vi "电源管理UI.vi"() -> ()   [LabVIEW 2016, in "PLC.lvlib"]
uses:
  PLC.lvlib
  <vilib>/Utility/miscctls.llb/LVPointTypeDef.ctl
panel:
  out "CODCr空闲时间":dbl caption="空闲时间:"
  out "总磷总氮空闲时间":dbl caption="空闲时间:"
  out "营养盐空闲时间":dbl caption="空闲时间:"
  out "CODMn空闲时间":dbl caption="空闲时间:"
  out "多参数空闲时间":dbl caption="空闲时间:"
  in  "CODCr电源":bool
  in  "总磷总氮电源":bool
  in  "营养盐电源":bool
  in  "CODMn电源":bool
  in  "多参数电源":bool
  # "说明：\n系统模式处于维护模式时，仪器电源自动打开；\n系统模式处于常规模式/质控模式/应急模式下，周期启动时，仪器电源自动打开；"
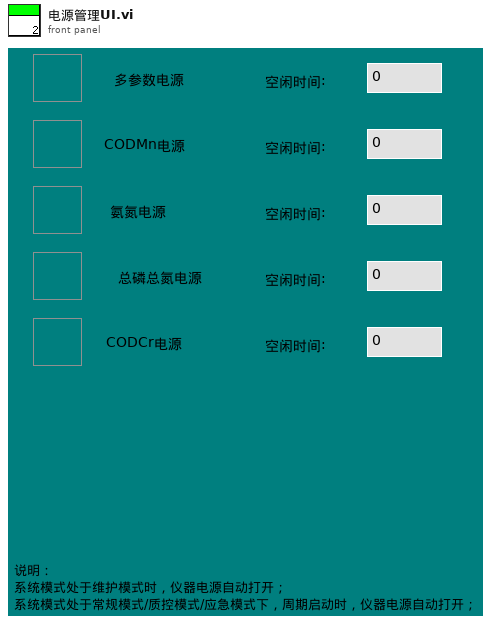
[diagram p1: front panel]
types:
  T1 = typedef "LVPointTypeDef.ctl" = cluster{"Horizontal":i16, "Vertical":i16}
  T2 = enum16{"空闲", "水样测试", "标样核查", "零点核查", "跨度核查", "空白测试", "平行样测试", "加标回收", "空白校准", "标样校准", "初始化（清洗）"}
  T3 = cluster{"R0":i16, "R1":i16, "R2":i16, "R3":i16, "R4":i16, "R5":i16, "R6":i16, "R7":i16, "R8":i16, "R9":i16, "R10":i16, "R11":i16, "R12":i16, "R13":i16, "R14":i16, "R15":i16, "R16":i16, "R17":i16, "R18":i16, "R19":i16, "R20":i16, "R21":i16, "R22":i16, "R23":i16, "R24":i16, "R25":i16, "R26":i16, "R27":i16, "R28":i16, "R29":i16, "R30":i16, "R31":i16, "R32":i16, "R33":i16, "R34":i16, "R35":i16, "R36":i16, "R37":i16, "R38":i16, "R39":i16, "R40":i16, "R41":i16, "R42":i16, "R43":i16, "R44":i16, "R45":i16, "R46":i16, "R47":i16, "R48":i16, "R49":i16, "R50":i16, "R51":i16, "R52":i16, "R53":i16, "R54":i16, "R55":i16, "R56":i16}
  T4 = cluster{"系统时间":timestamp, "工作状态":enum16{"空闲", "水样测试", "标样核查", "零点核查", "跨度核查", "空白测试", "平行样测试", "加标回收", "空白校准", "标样校准", "初始化（清洗）"}, "测量模式":enum16{"待机", "连续模式", "周期模式", "定点模式", "受控模式", "手动模式"}, "告警代码":enum16{"无告警", "缺试剂告警", "缺水样告警", "缺蒸馏水告警", "缺标液告警", "仪表漏液告警", "标定异常告警", "超量程告警", "加热异常", "低试剂预警", "超上限告警", "超下限告警", "仪表内部其他异常", "滴定异常告警", "电极异常告警", "量程切换告警", "参数设置告警", "PH电极电位异常", "电导率电极异常", "浊度光度异常", "溶解氧电极异常", "溶解氧光强异常", "温度异常告警", "PH异常告警", "溶解氧异常告警", "电导率异常告警", "浊度异常告警", "叶绿素异常告警", "藻密度异常告警", "蓝绿藻异常告警", "ORP异常告警", "氨氮异常告警", "清洁刷异常告警", "SD卡异常告警", "蓝牙异常告警", "Wifi异常告警", "流程异常告警"}, "故障代码":enum16{"无故障", "电机故障", "温度故障", "通讯故障", "滴定故障"}, "日志代码":u16, "软件版本":u16, "F0":sgl, "F1":sgl, "F2":sgl, "F3":sgl, "T":sgl, "H":sgl, "id":u16, "flowid":u16, "量程":u16, "总磷控温温度1":sgl, "营养盐控温温度2":sgl, "ADC":sgl}
  T5 = cluster{"系统时间":timestamp, "工作状态":u16, "测量模式":u16, "告警代码":enum16{"无告警", "缺试剂告警", "缺水样告警", "缺蒸馏水告警", "缺标液告警", "仪表漏液告警", "标定异常告警", "超量程告警", "加热异常", "低试剂预警", "超上限告警", "超下限告警", "仪表内部其他异常", "滴定异常告警", "电极异常告警", "量程切换告警", "参数设置告警", "PH电极电位异常", "电导率电极异常", "浊度光度异常", "溶解氧电极异常", "溶解氧光强异常", "温度异常告警", "PH异常告警", "溶解氧异常告警", "电导率异常告警", "浊度异常告警", "叶绿素异常告警", "藻密度异常告警", "蓝绿藻异常告警", "ORP异常告警", "氨氮异常告警", "清洁刷异常告警", "SD卡异常告警", "蓝牙异常告警", "Wifi异常告警", "流程异常告警"}, "故障代码":enum16{"无故障", "电机故障", "温度故障", "通讯故障", "滴定故障"}, "日志代码":u16, "软件版本":string}
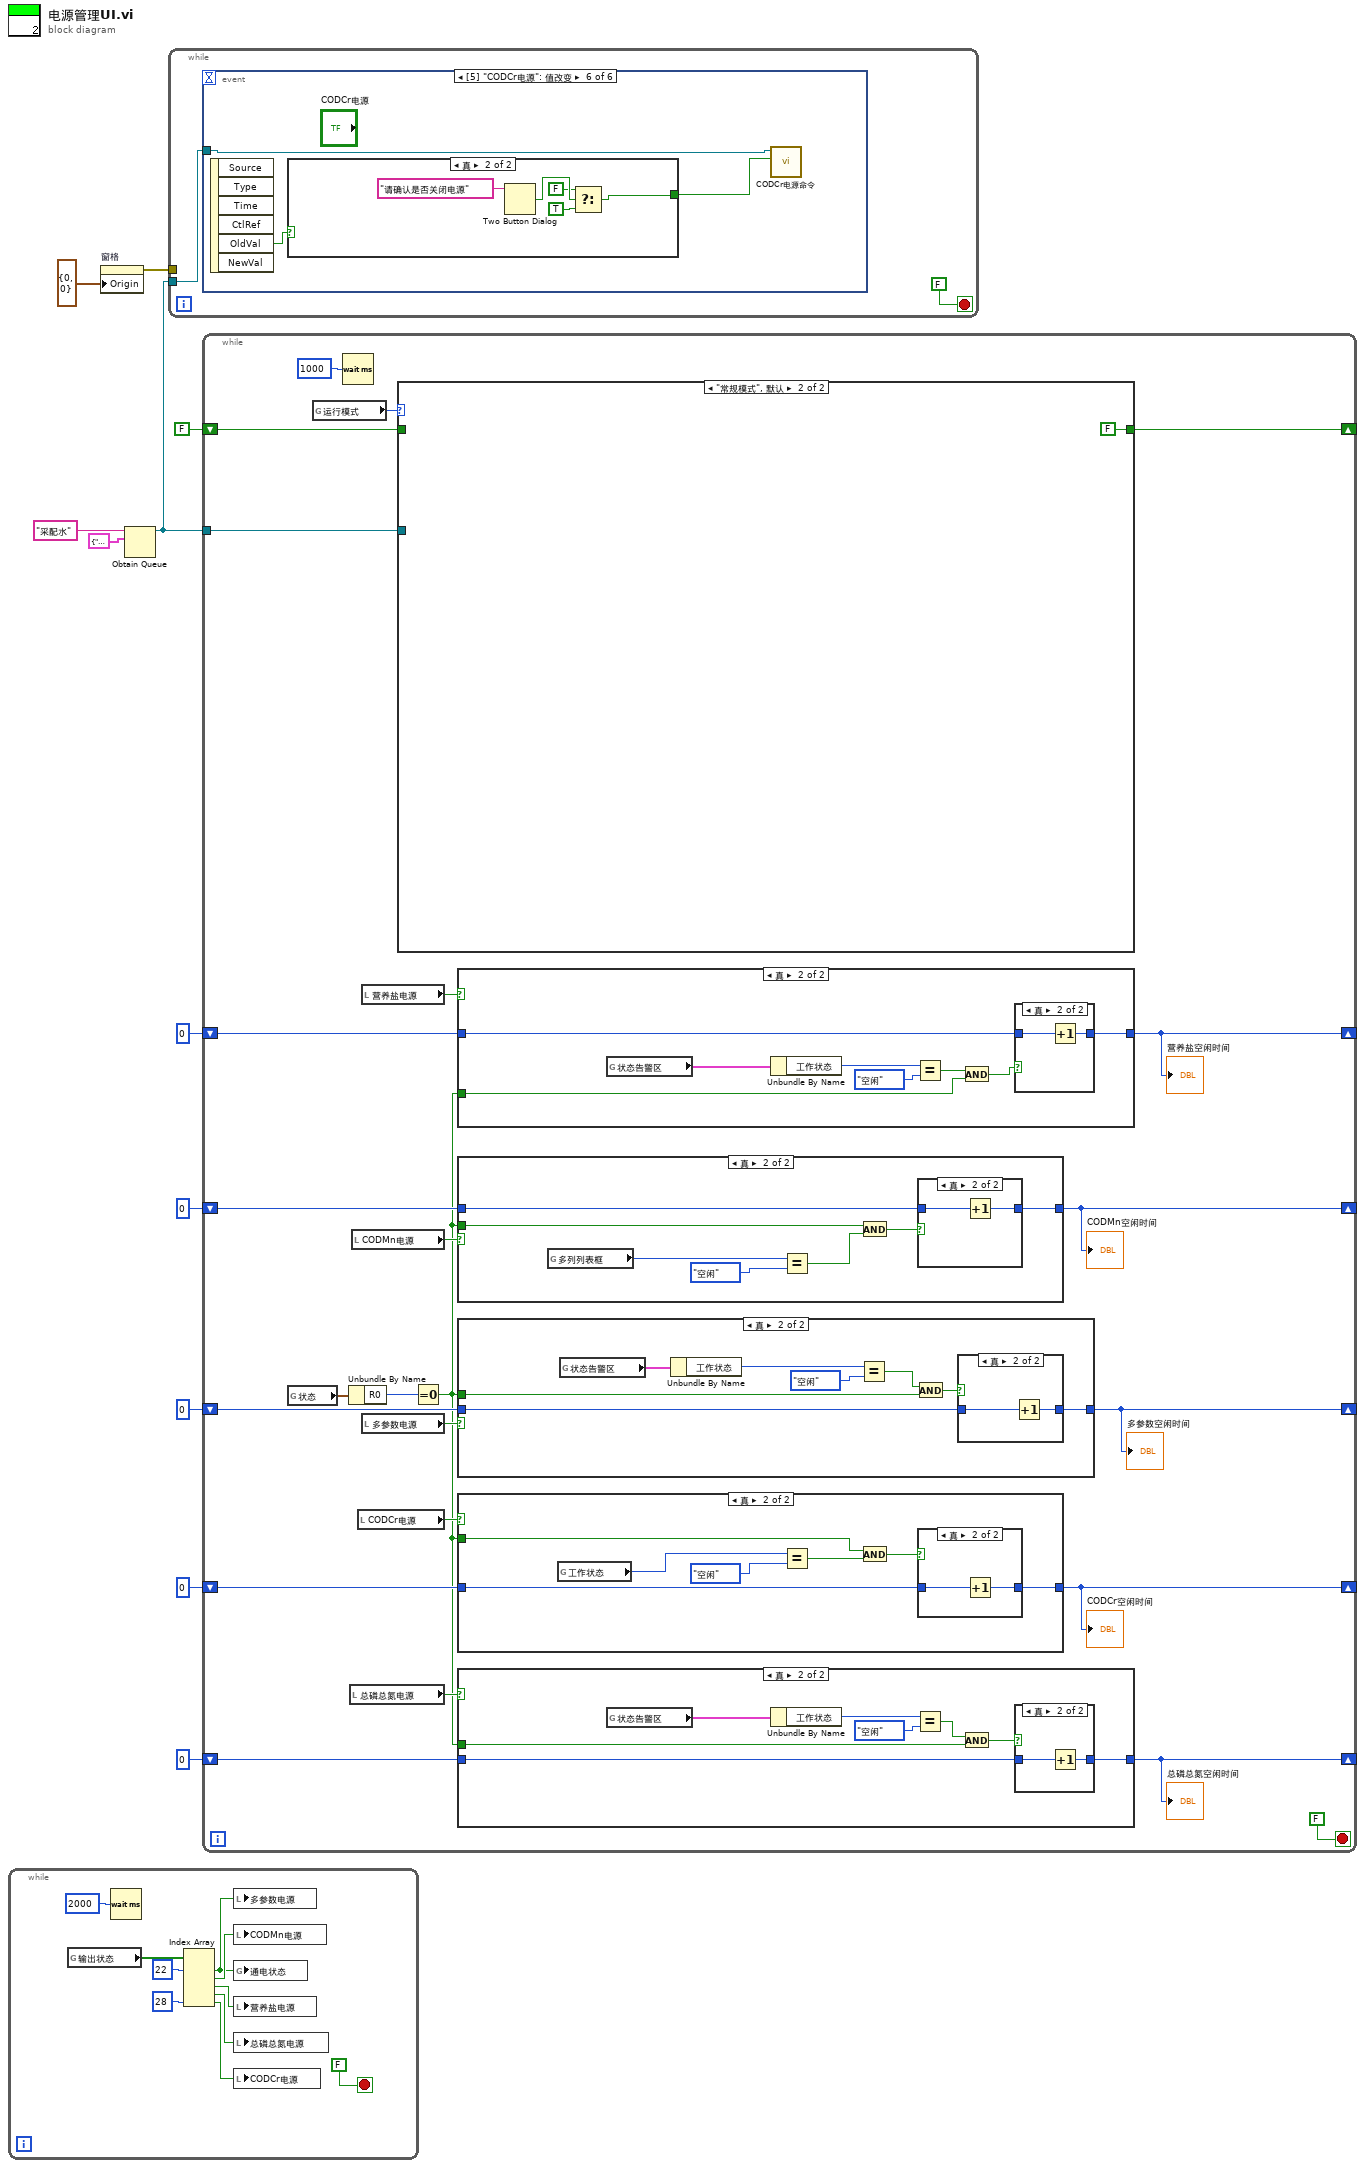
[diagram p0: block diagram]
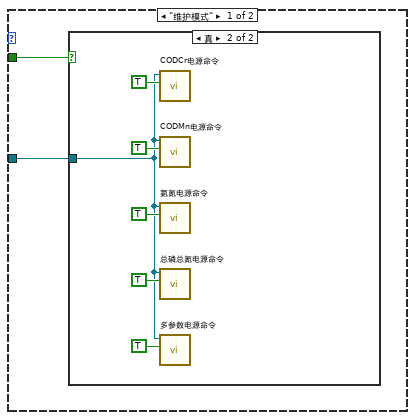
[diagram p2: hidden frame]
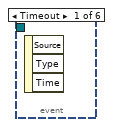
[diagram p14: hidden frame]
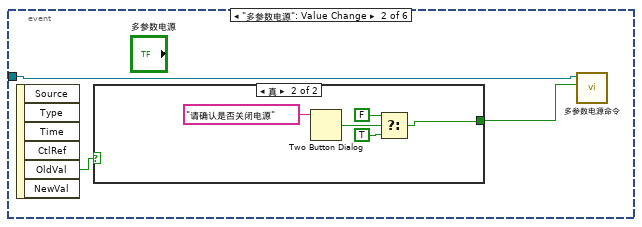
[diagram p15: hidden frame]
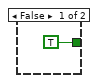
[diagram p16: hidden frame]
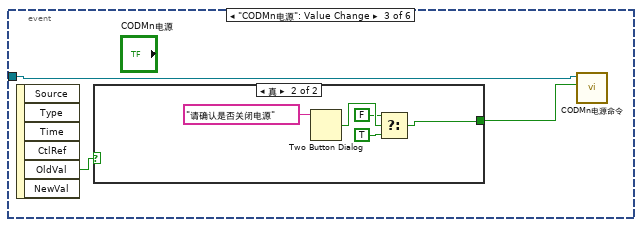
[diagram p17: hidden frame]
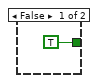
[diagram p18: hidden frame]
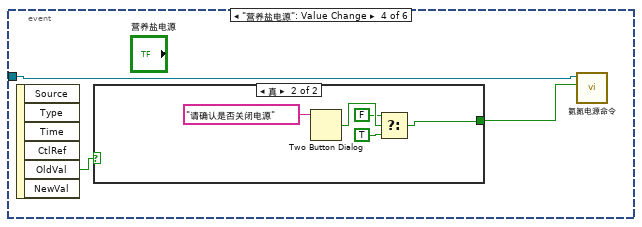
[diagram p19: hidden frame]
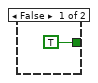
[diagram p20: hidden frame]
diagram:
  n1 = while {
    stop <- FALSE stop-if-true
    n2 = global read "采配水全局变量.vi" "输出状态"() -> (w19:bool[])
    n3 = Wait (ms)(milliseconds to wait=u32 2000 ("等待时间（毫秒）")) -> ()  [unwired: 1 out]
    n4 = Index Array(array=w19, index #1=22 ("索引"), index #5=28 ("索引")) -> (element #1=w14:bool, element #2=w17:bool, element #3=w16:bool, element #4=w15:bool, element #5=w13:bool)  [unwired: 3 in]
    n5 = local write "多参数电源"(w14) -> ()
    n6 = local write "CODMn电源"(w17) -> ()
    n7 = global write "多参数全局变量.vi" "通电状态"(w14) -> ()
    n8 = local write "营养盐电源"(w16) -> ()
    n9 = local write "总磷总氮电源"(w15) -> ()
    n10 = local write "CODCr电源"(w13) -> ()
  }
  n11 = property on="窗格" class="Pane"("Origin"=T1 {"Horizontal"=0, "Vertical"=0} ("原点")) -> (error out=w8:errorcluster)  [unwired: 2 in, 1 out]
  n12 = Obtain Queue(name (unnamed)="采配水" ("名称（未命名）"), element data type=cluster{"命令":string, "数据":variant} {"命令"="", "数据"=variant}) -> (queue out=w7:refnum<queue>)  [unwired: 3 in, 2 out]
  n13 = while {
    tunnel: w7 -> [w22]
    tunnel: w8 -> [_]
    stop <- FALSE stop-if-true
    n14 = event shown="[5] \"CODCr电源\": 值改变" {
      selector: _ -> [_ _ _ _ _ _]
      dyn-events: _ -> [_ _ _ _ _ _]
      timeout: _ -> [_ _ _ _ _ _]
      tunnel: w22 -> [_ w26 w35 w44 w53 w62]
      event Timeout {
        n15 = event-data() -> ()  [unwired: 1 in, 3 out]
      }
      event "多参数电源": Value Change {
        n16 = event-data() -> ("OldVal"=w25:bool)  [unwired: 1 in, 5 out]
        n17 = case shown="真" w25 {
          tunnel: [TRUE ("T button?") w28] -> w24
          frame False {
          }
          frame True {
            n18 = Two Button Dialog(message="请确认是否关闭电源" ("消息")) -> (T button?=w31:bool)  [unwired: 2 in]
            n19 = Select(t=FALSE, s=w31, f=TRUE ("T button?")) -> (s? t:f=w28:bool)
          }
        }
        n20 = call "多参数电源命令.vi"("通电/断电"=w24, "队列"=w26) -> ()  [unwired: 9 in, 1 out]
      }
      event "CODMn电源": Value Change {
        n21 = event-data() -> ("OldVal"=w34:bool)  [unwired: 1 in, 5 out]
        n22 = case shown="真" w34 {
          tunnel: [TRUE ("T button?") w37] -> w33
          frame False {
          }
          frame True {
            n23 = Two Button Dialog(message="请确认是否关闭电源" ("消息")) -> (T button?=w40:bool)  [unwired: 2 in]
            n24 = Select(t=FALSE, s=w40, f=TRUE ("T button?")) -> (s? t:f=w37:bool)
          }
        }
        n25 = call "CODMn电源命令.vi"("通电/断电"=w33, "队列"=w35) -> ()  [unwired: 9 in, 1 out]
      }
      event "营养盐电源": Value Change {
        n26 = event-data() -> ("OldVal"=w43:bool)  [unwired: 1 in, 5 out]
        n27 = case shown="真" w43 {
          tunnel: [TRUE ("T button?") w46] -> w42
          frame False {
          }
          frame True {
            n28 = Two Button Dialog(message="请确认是否关闭电源" ("消息")) -> (T button?=w49:bool)  [unwired: 2 in]
            n29 = Select(t=FALSE, s=w49, f=TRUE ("T button?")) -> (s? t:f=w46:bool)
          }
        }
        n30 = call "氨氮电源命令.vi"("通电/断电"=w42, "队列"=w44) -> ()  [unwired: 9 in, 1 out]
      }
      event "总磷总氮电源": Value Change {
        n31 = event-data() -> ("OldVal"=w52:bool)  [unwired: 1 in, 5 out]
        n32 = case shown="真" w52 {
          tunnel: [TRUE ("T button?") w55] -> w51
          frame False {
          }
          frame True {
            n33 = Two Button Dialog(message="请确认是否关闭电源" ("消息")) -> (T button?=w58:bool)  [unwired: 2 in]
            n34 = Select(t=FALSE, s=w58, f=TRUE ("T button?")) -> (s? t:f=w55:bool)
          }
        }
        n35 = call "总磷总氮电源命令.vi"("通电/断电"=w51, "队列"=w53) -> ()  [unwired: 9 in, 1 out]
      }
      event "CODCr电源": Value Change {
        n36 = event-data() -> ("OldVal"=w61:bool)  [unwired: 1 in, 5 out]
        n37 = case shown="真" w61 {
          tunnel: [TRUE ("T button?") w64] -> w60
          frame False {
          }
          frame True {
            n38 = Two Button Dialog(message="请确认是否关闭电源" ("消息")) -> (T button?=w67:bool)  [unwired: 2 in]
            n39 = Select(t=FALSE, s=w67, f=TRUE ("T button?")) -> (s? t:f=w64:bool)
          }
        }
        n40 = call "CODCr电源命令.vi"("通电/断电"=w60, "队列"=w62) -> ()  [unwired: 9 in, 1 out]
      }
    }
  }
  n41 = while {
    tunnel: w7 -> [w75]
    shift-right: [w76] -> _
    shift-left: u32 0 ("等待时间（毫秒）") -> [w89]
    shift-right: [w80] -> _
    shift-left: u32 0 ("等待时间（毫秒）") -> [w87]
    shift-right: [w78] -> _
    shift-left: u32 0 ("等待时间（毫秒）") -> [w83]
    shift-right: [w79] -> _
    shift-left: u32 0 ("等待时间（毫秒）") -> [w84]
    shift-right: [w77] -> _
    shift-left: u32 0 ("等待时间（毫秒）") -> [w82]
    shift-right: [w72] -> _
    shift-left: FALSE -> [w73]
    stop <- FALSE stop-if-true
    n42 = global read "采配水全局变量.vi" "状态"() -> (w71:T3)
    n43 = global read "系统变量.vi" "运行模式"() -> (w74:enum16{"维护模式", "常规模式", "应急模式", "质控模式"})
    n44 = Wait (ms)(milliseconds to wait=u32 1000 ("等待时间（毫秒）")) -> ()  [unwired: 1 out]
    n45 = Unbundle By Name(w71) -> ("R0"=w70:i16)
    n46 = local read "总磷总氮电源"() -> (w86:bool)
    n47 = local read "CODMn电源"() -> (w88:bool)
    n48 = local read "CODCr电源"() -> (w81:bool)
    n49 = local read "营养盐电源"() -> (w90:bool)
    n50 = local read "多参数电源"() -> (w85:bool)
    n51 = case shown="\"常规模式\", 默认" w74 {
      tunnel: w75 -> [w94 _]
      tunnel: w73 -> [w93 _]
      tunnel: [_ FALSE] -> w72
      frame "维护模式" {
        n52 = case shown="真" w93 {
          tunnel: w94 -> [_ w95]
          frame False {
          }
          frame True {
            n53 = call "CODCr电源命令.vi"("通电/断电"=TRUE, "队列"=w95) -> ()  [unwired: 9 in, 1 out]
            n54 = call "CODMn电源命令.vi"("通电/断电"=TRUE, "队列"=w95) -> ()  [unwired: 9 in, 1 out]
            n55 = call "氨氮电源命令.vi"("通电/断电"=TRUE, "队列"=w95) -> ()  [unwired: 9 in, 1 out]
            n56 = call "总磷总氮电源命令.vi"("通电/断电"=TRUE, "队列"=w95) -> ()  [unwired: 9 in, 1 out]
            n57 = call "多参数电源命令.vi"("通电/断电"=TRUE, "队列"=w95) -> ()  [unwired: 9 in, 1 out]
          }
        }
      }
      frame "常规模式", Default {
      }
    }
    n58 = Equal To 0?(x=w70) -> (x = 0?=w69:bool)
    n59 = case shown="真" w90 {
      tunnel: w89 -> [_ w147]
      tunnel: [_ w143] -> w76
      tunnel: w69 -> [_ w140]
      frame False {
      }
      frame True {
        n60 = global read "VAR氨氮全局变量.vi" "状态告警区"() -> (w142:T4)
        n61 = Unbundle By Name(w142) -> ("工作状态"=w146:T2)
        n62 = Equal?(x=w146, y=T2."空闲" ("工作状态")) -> (x = y?=w144:bool)
        n63 = And(x=w144, y=w140) -> (x .and. y?=w141:bool)
        n64 = case shown="真" w141 {
          tunnel: w147 -> [_ w149]
          tunnel: [_ w148] -> w143
          frame False {
          }
          frame True {
            n65 = Increment(x=w149) -> (x+1=w148:u32)
          }
        }
      }
    }
    "营养盐空闲时间" <- w76
    n66 = case shown="真" w88 {
      tunnel: w87 -> [_ w137]
      tunnel: [_ w134] -> w80
      tunnel: w69 -> [_ w131]
      frame False {
      }
      frame True {
        n67 = global read "运行时序全局变量.vi" "多列列表框"() -> (w133:i32)
        n68 = Equal?(x=w133, y=T2."空闲" ("工作状态")) -> (x = y?=w135:bool)
        n69 = And(x=w131, y=w135) -> (x .and. y?=w132:bool)
        n70 = case shown="真" w132 {
          tunnel: w137 -> [_ w139]
          tunnel: [_ w138] -> w134
          frame False {
          }
          frame True {
            n71 = Increment(x=w139) -> (x+1=w138:u32)
          }
        }
      }
    }
    "CODMn空闲时间" <- w80
    n72 = case shown="真" w85 {
      tunnel: w83 -> [_ w118]
      tunnel: [_ w115] -> w78
      tunnel: w69 -> [_ w111]
      frame False {
      }
      frame True {
        n73 = global read "多参数全局变量.vi" "状态告警区"() -> (w114:T5)
        n74 = Unbundle By Name(w114) -> ("工作状态"=w113:u16)
        n75 = Equal?(x=w113, y=T2."空闲" ("工作状态")) -> (x = y?=w116:bool)
        n76 = And(x=w116, y=w111) -> (x .and. y?=w112:bool)
        n77 = case shown="真" w112 {
          tunnel: w118 -> [_ w120]
          tunnel: [_ w119] -> w115
          frame False {
          }
          frame True {
            n78 = Increment(x=w120) -> (x+1=w119:u32)
          }
        }
      }
    }
    "多参数空闲时间" <- w78
    n79 = case shown="真" w81 {
      tunnel: w82 -> [_ w108]
      tunnel: [_ w105] -> w77
      tunnel: w69 -> [_ w102]
      frame False {
      }
      frame True {
        n80 = global read "CODcr全局变量.vi" "工作状态"() -> (w104:T2)
        n81 = Equal?(x=w104, y=T2."空闲" ("工作状态")) -> (x = y?=w106:bool)
        n82 = And(x=w102, y=w106) -> (x .and. y?=w103:bool)
        n83 = case shown="真" w103 {
          tunnel: w108 -> [_ w110]
          tunnel: [_ w109] -> w105
          frame False {
          }
          frame True {
            n84 = Increment(x=w110) -> (x+1=w109:u32)
          }
        }
      }
    }
    "CODCr空闲时间" <- w77
    n85 = case shown="真" w86 {
      tunnel: w84 -> [_ w128]
      tunnel: [_ w125] -> w79
      tunnel: w69 -> [_ w121]
      frame False {
      }
      frame True {
        n86 = global read "VAR总磷总氮全局变量.vi" "状态告警区"() -> (w124:T4)
        n87 = Unbundle By Name(w124) -> ("工作状态"=w123:T2)
        n88 = Equal?(x=w123, y=T2."空闲" ("工作状态")) -> (x = y?=w126:bool)
        n89 = And(x=w126, y=w121) -> (x .and. y?=w122:bool)
        n90 = case shown="真" w122 {
          tunnel: w128 -> [_ w130]
          tunnel: [_ w129] -> w125
          frame False {
          }
          frame True {
            n91 = Increment(x=w130) -> (x+1=w129:u32)
          }
        }
      }
    }
    "总磷总氮空闲时间" <- w79
  }
